vi "xiCam - CloseDevice.vi"(8 "error in (no error)":errorcluster, 11 "xiCam In":refnum<k24>) -> (0 "error out":errorcluster)   [LabVIEW 2015]
doc: "This function uninitializes the specified device and releases allocated resources.\n\n<b>void CloseDevice()</b>"
uses:
  C:/GIT/Cameras3.x/Integrations/Labview/xiLib/xiLIB_32bit/xiLIB/xiCamLib/API/x86/xiApi.NET.dll
  xiLIB_32bit/xiLIB/xiCamLib/API/x86/xiApi.NET.dll
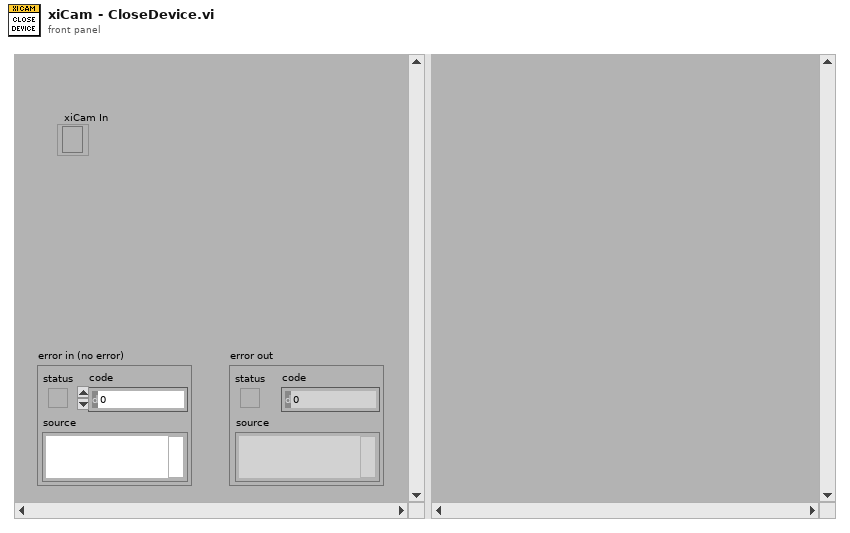
[diagram p1: front panel]
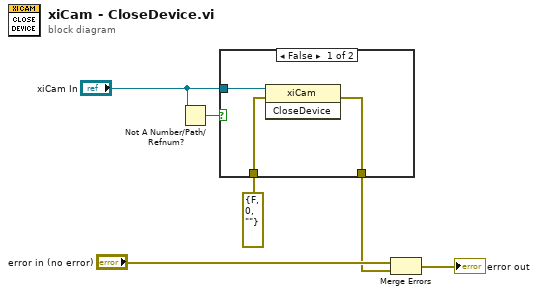
[diagram p0: block diagram]
diagram:
  n1 = Not A Number/Path/Refnum?(number/path/refnum="xiCam In") -> (NaN/Path/Refnum?=w5:bool)
  n2 = case shown="False" w5 {
    tunnel: errorcluster {"status"=FALSE, "code"=0, "source"=""} ("error in (no error) 2") -> [w9 w10]
    tunnel: [w8 w10] -> w2
    tunnel: "xiCam In" -> [w7 _]
    frame False {
      n3 = invoke class="xiCam" method="CloseDevice"(reference=w7, error in=w9) -> (error out=w8:errorcluster)  [unwired: 1 in, 2 out]
    }
    frame True {
    }
  }
  n4 = Merge Errors("error in (no error)", w2) -> (→"error out":errorcluster)
